vi "Configure Vacuum Setting.vi"(8 "error in (no error)":errorcluster, 10 "Vacuum Setting (0000)":i64 min=0 max=1000 step=1 format="%04.0f", 11 "VISA resource name":refnum<visa-resource-name>) -> (0 "error out":errorcluster, 3 "VISA resource name out":refnum<visa-resource-name>)   [LabVIEW 2018, in "EFD Ultimus V.lvlib"]
doc: "This vi updates the vaccum value in the current memory location.\n\nHost Format: VS--vvvv\nWhere\n-- :two spaces\nvvvv:The 4-digit vacuum,setting excluding the decimal point. This is a unitless value. The valid vacuum ranges and decimal point are determined by the vacuum units currently selected in the dispenser."
uses:
  EFD Ultimus V.lvlib
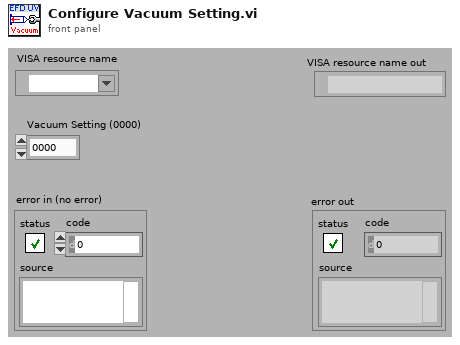
[diagram p1: front panel]
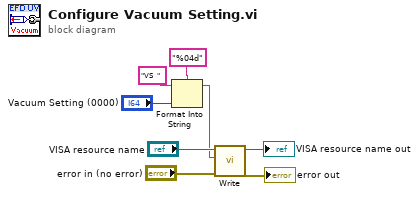
[diagram p0: block diagram]
diagram:
  n1 = Format Into String(format string="%04d", initial string="VS  " ("string"), "Vacuum Setting (0000)") -> (resulting string=w4:string)  [unwired: 1 in, 1 out]
  n2 = call "Write.vi"("error in (no error)"="error in (no error)", "Command To Write"=w4, "VISA resource name"="VISA resource name") -> ("error out"=→"error out":errorcluster, "VISA resource name out"=→"VISA resource name out":refnum<visa-resource-name>)  [unwired: 7 out]
